vi "betav3 labview.vi"() -> ()   [LabVIEW 2016]
uses:
  <vilib>/Instr/_visa.llb/VISA Configure Serial Port (Instr).vi
panel:
  in  "Stop":bool
  out "Arduino connecté ?":bool
  in  "Port de communication":refnum<visa-resource-name>="COM4"
  in  "?":T1(tab)
  in  "Emplacement mémoire":string(combo)
  out "Données lue":string
  in  "Adresse de fin+1":string
  in  "Adresse de début":string
  in  "Données à écrire":string
  in  "Lecture":bool
  in  "Ecriture":bool
  in  "Lecture totale de l'EEPROM":bool
  out "Commentaire 2":string
  out "Board serial number":string
  out "Code article":string
  out "Test sonde mobile":string
  out "Test synor":string
  out "Test ICT":string
  out "Test FCT1":string
  out "Test ESS":string
  out "Test FCT2":string
  out "Version soft 1":string
  out "Version soft 2":string
  out "Commentaires 1":string
  out "Version soft 3":string
  out "Mapping":string
  # "Programmateur EEPROM beta v2"
  # "Programmateur EEPROM"
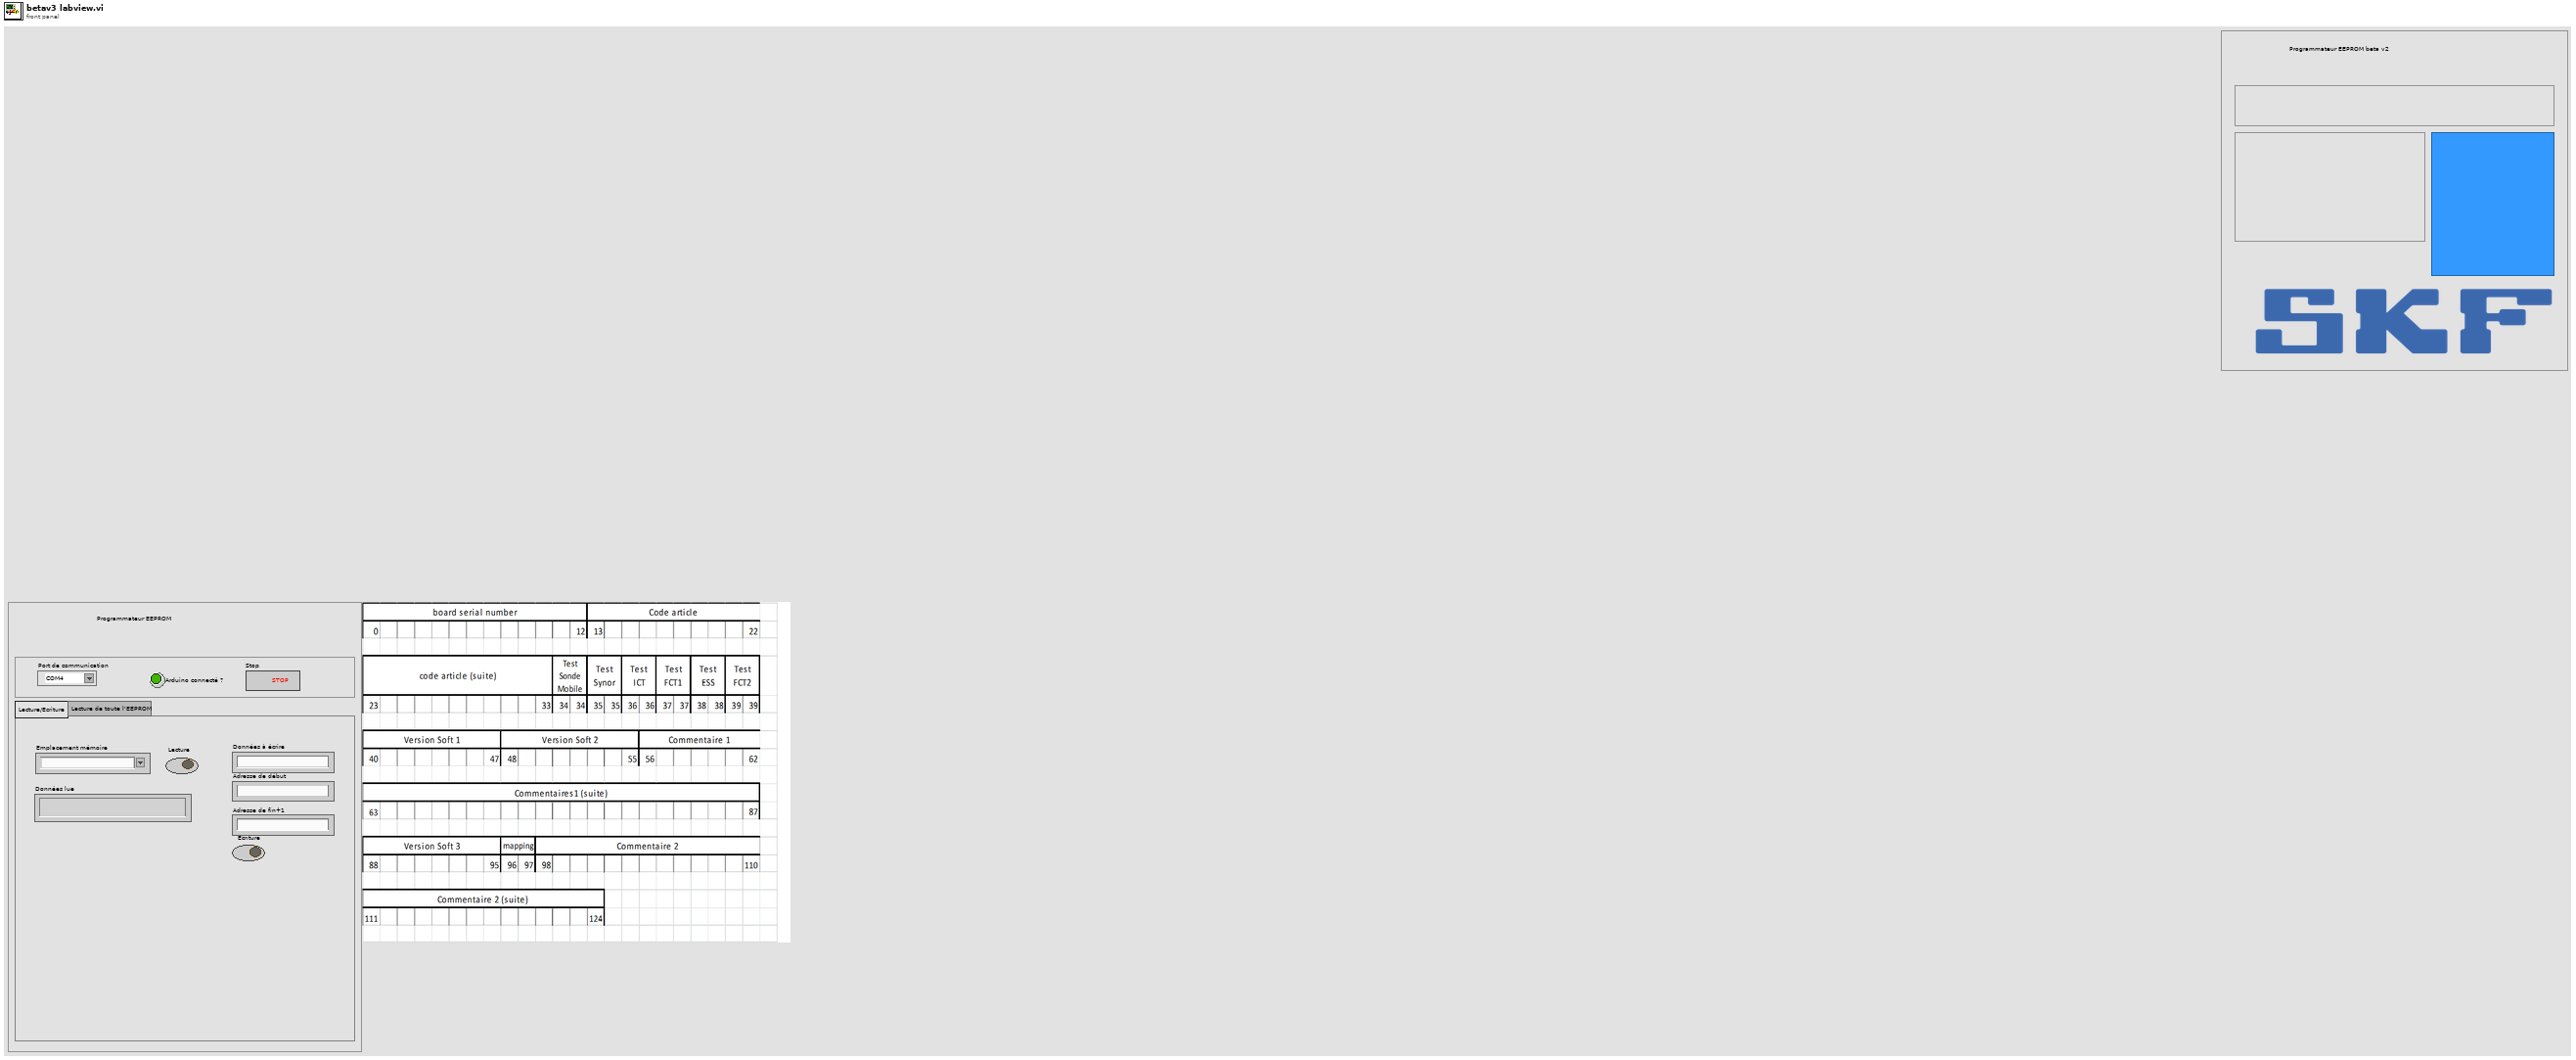
[diagram p1: front panel]
types:
  T1 = enum32{"Lecture/Ecriture", "Lecture de toute l'EEPROM"}
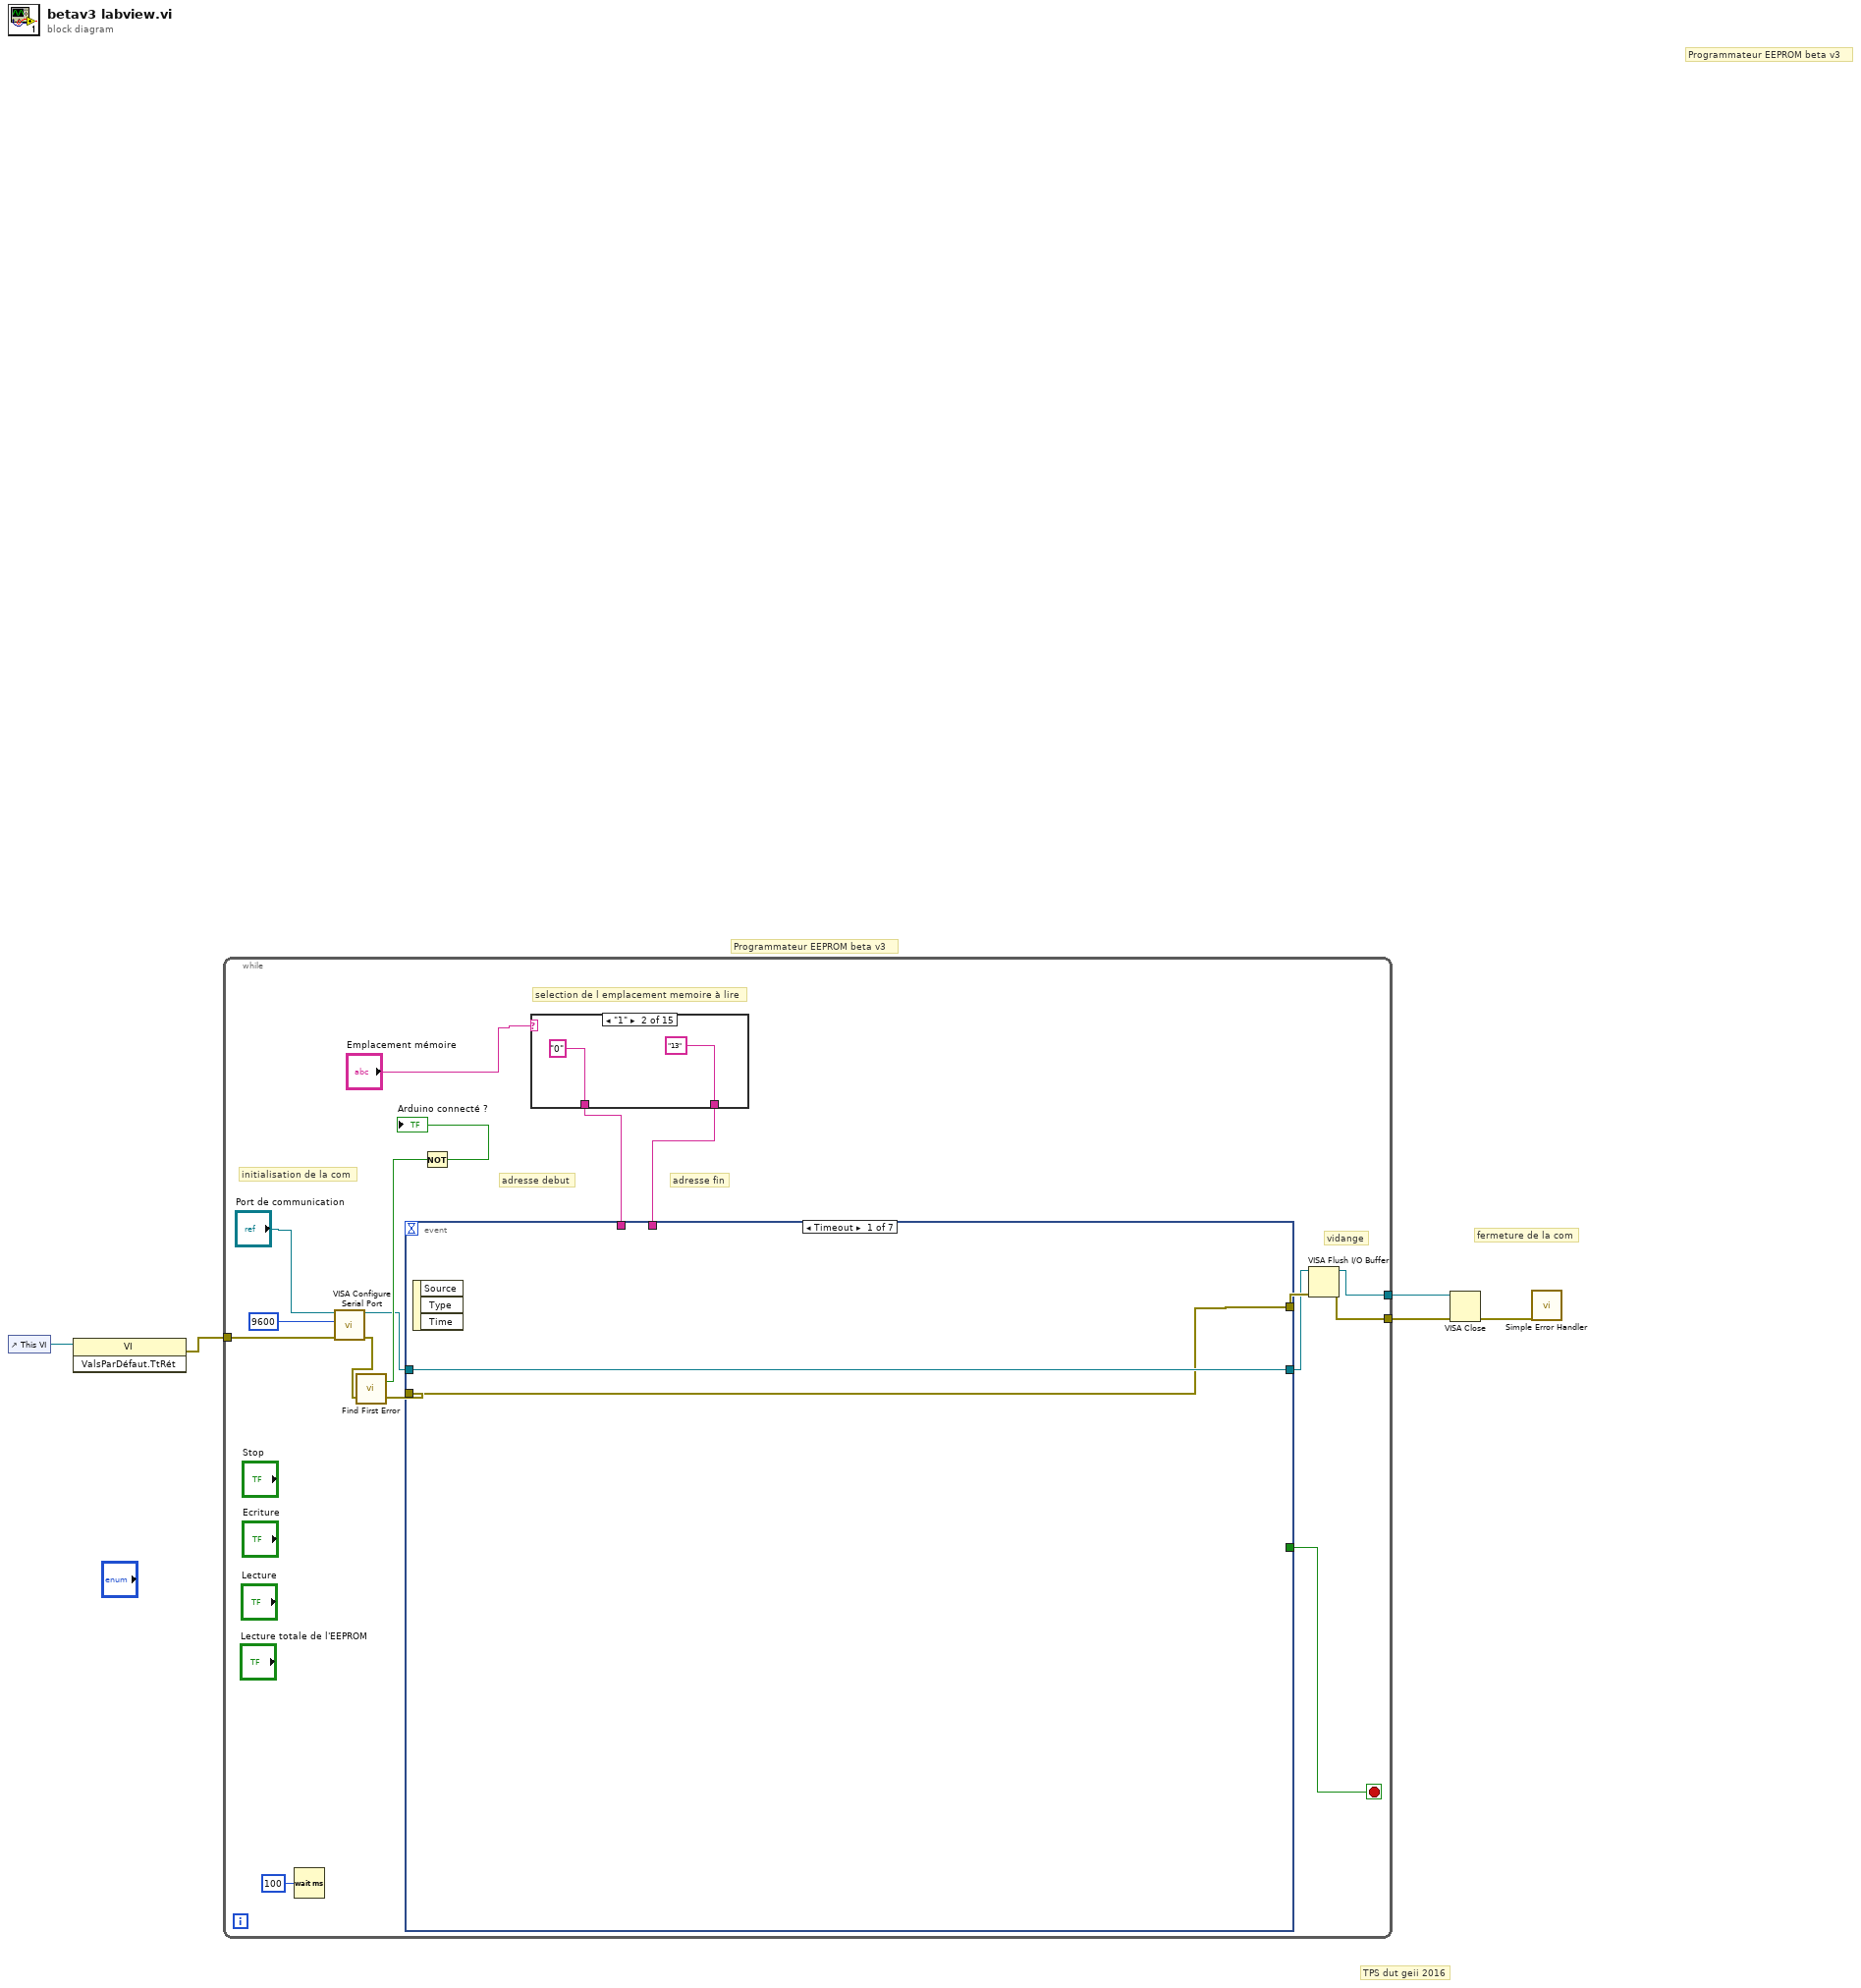
[diagram p0: block diagram]
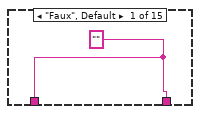
[diagram p2: hidden frame]
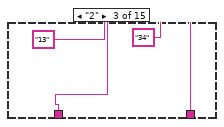
[diagram p3: hidden frame]
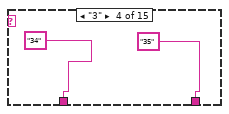
[diagram p4: hidden frame]
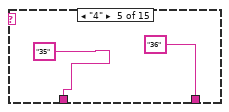
[diagram p5: hidden frame]
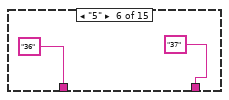
[diagram p6: hidden frame]
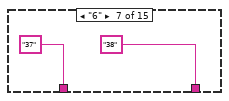
[diagram p7: hidden frame]
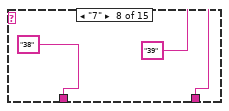
[diagram p8: hidden frame]
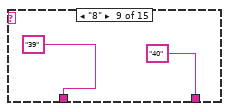
[diagram p9: hidden frame]
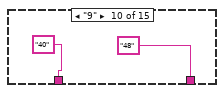
[diagram p10: hidden frame]
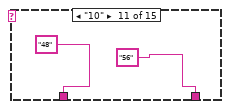
[diagram p11: hidden frame]
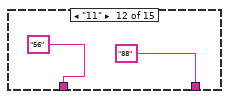
[diagram p12: hidden frame]
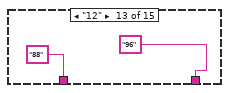
[diagram p13: hidden frame]
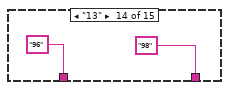
[diagram p14: hidden frame]
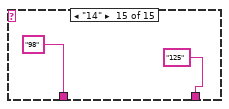
[diagram p15: hidden frame]
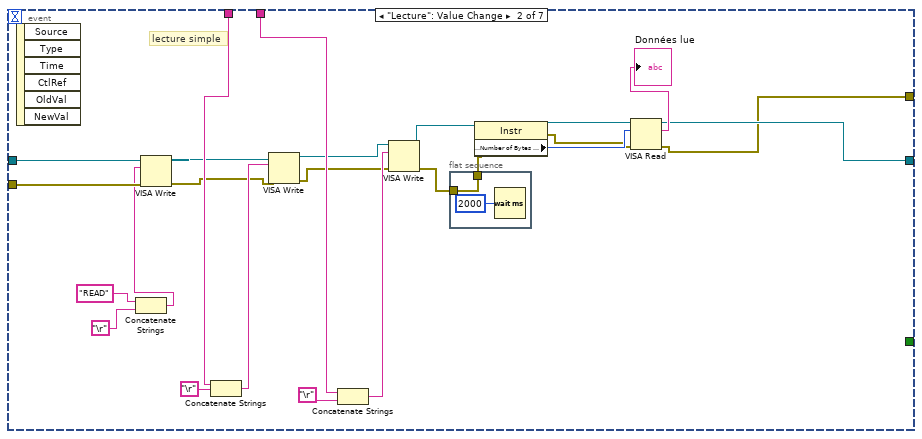
[diagram p16: hidden frame]
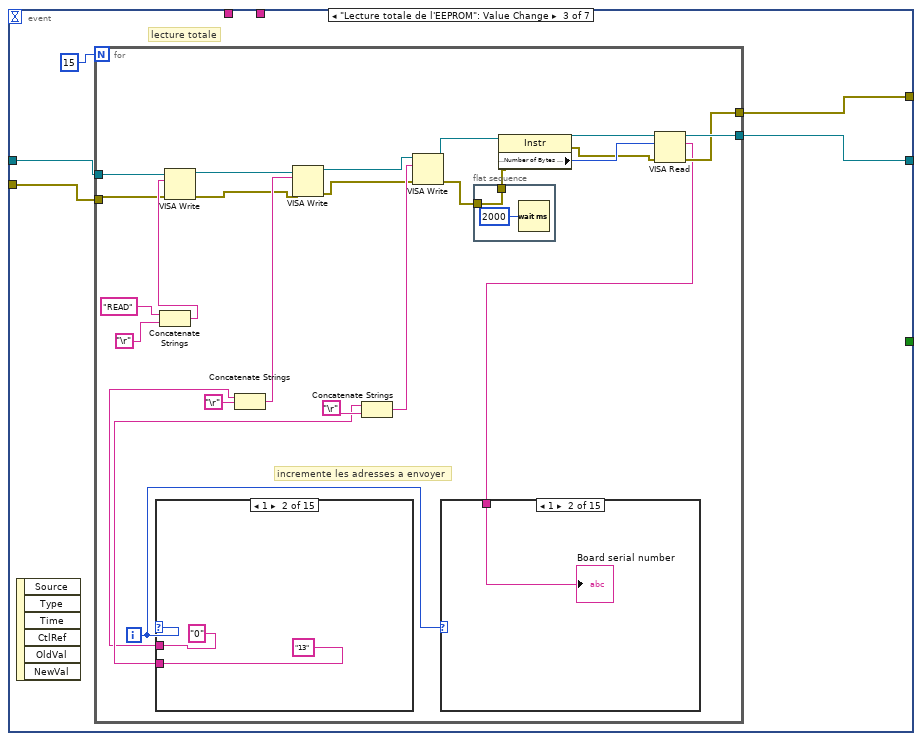
[diagram p17: hidden frame]
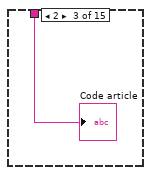
[diagram p19: hidden frame]
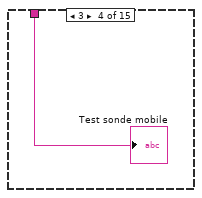
[diagram p20: hidden frame]
diagram:
  # "fermeture de la com"
  # "TPS dut geii 2016"
  # "Programmateur EEPROM beta v3"
  # "Programmateur EEPROM beta v3"
  n1 = control-ref of="This VI"() -> (w4:refnum<vi>)
  n2 = invoke class="VI" method="ValsParDéfaut.TtRét"(reference=w4) -> (error out=w1:errorcluster)  [unwired: 2 in, 2 out]
  n3 = while {
    tunnel: [w17] -> w5
    tunnel: [w16] -> w3
    tunnel: w1 -> [w15]
    stop <- w8 stop-if-true
    # "vidange"
    # "selection de l emplacement memoire à lire"
    # "initialisation de la com"
    # "adresse fin"
    # "adresse debut"
    n4 = Wait (ms)(milliseconds to wait=u32 100 ("attente (ms)")) -> ()  [unwired: 1 out]
    n5 = call-poly "VISA Configure Serial Port"("VISA resource name"="Port de communication", "baud rate (9600)"=u32 9600, "error in (no error)"=w15) -> ("VISA resource name out"=w13:refnum<visa-resource-name>, "error out"=w14:errorcluster)  [unwired: 11 in]
    n6 = call <vilib>:"Find First Error.vi"("error in (no error)"=w14) -> ("error out"=w18:errorcluster, "error?"=w19:bool)  [unwired: 3 in]
    n7 = Not(x=w19) -> (.not. x?=→"Arduino connecté ?":bool)
    n8 = case shown="\"1\"" "Emplacement mémoire" {
      tunnel: [w23 "0" "13" "34" "35" "36" "37" "38" "39" "40" "48" "56" "88" "96" "98"] -> w10
      tunnel: [w23 "13" "34" "35" "36" "37" "38" "39" "40" "48" "56" "88" "96" "98" "125"] -> w9
      frame "Faux", Default {
        w23 = ""
      }
      frame "1" {
      }
      frame "2" {
      }
      frame "3" {
      }
      frame "4" {
      }
      frame "5" {
      }
      frame "6" {
      }
      frame "7" {
      }
      frame "8" {
      }
      frame "9" {
      }
      frame "10" {
      }
      frame "11" {
      }
      frame "12" {
      }
      frame "13" {
      }
      frame "14" {
      }
    }
    n9 = event shown="[0] Timeout" {
      selector: _ -> [_ _ _ _ _ _ _]
      dyn-events: _ -> [_ _ _ _ _ _ _]
      timeout: _ -> [_ _ _ _ _ _ _]
      tunnel: w13 -> [w53 w77 w84 w155 w157 w159 w170]
      tunnel: w10 -> [_ w76 _ _ _ _ _]
      tunnel: w9 -> [_ w75 _ _ _ _ _]
      tunnel: w18 -> [w52 w74 w83 w156 w158 w160 w169]
      tunnel: [_ _ _ _ _ TRUE _] -> w8
      tunnel: [w53 w55 w82 w155 w157 w159 w164] -> w6
      tunnel: [w52 w54 w81 w156 w158 w160 w162] -> w7
      event Timeout {
        n10 = event-data() -> ()  [unwired: 1 in, 3 out]
      }
      event "Lecture": Value Change {
        # "lecture simple"
        n11 = event-data() -> ()  [unwired: 1 in, 6 out]
        n12 = Concatenate Strings("READ", "\r") -> (w70:string)
        n13 = VISA Write(VISA resource name=w77, write buffer=w70, error in (no error)=w74) -> (VISA resource name out=w69:refnum<visa-resource-name>, error out=w60:errorcluster)  [unwired: 1 out]
        n14 = Concatenate Strings(w76, "\r") -> (w67:string)
        n15 = VISA Write(VISA resource name=w69, write buffer=w67, error in (no error)=w60) -> (VISA resource name out=w66:refnum<visa-resource-name>, error out=w59:errorcluster)  [unwired: 1 out]
        n16 = Concatenate Strings(w75, "\r") -> (w64:string)
        n17 = VISA Write(VISA resource name=w66, write buffer=w64, error in (no error)=w59) -> (VISA resource name out=w61:refnum<visa-resource-name>, error out=w56:errorcluster)  [unwired: 1 out]
        n18 = flat-sequence {
          tunnel: [w78] -> w57
          tunnel: w56 -> [w78]
          frame #0 {
            n19 = Wait (ms)(milliseconds to wait=u32 2000 ("attente (ms)")) -> ()  [unwired: 1 out]
          }
        }
        n20 = property class="Instr"(reference=w61, error in=w57) -> (reference out=w62:refnum<visa-resource-name>, error out=w58:errorcluster, "Serial Settings:Number of Bytes at Serial Port"=w63:u32)
        n21 = VISA Read(VISA resource name=w62, byte count=w63, error in (no error)=w58) -> (VISA resource name out=w55:refnum<visa-resource-name>, read buffer=→"Données lue":string, error out=w54:errorcluster)  [unwired: 1 out]
      }
      event "Lecture totale de l'EEPROM": Value Change {
        # "lecture totale"
        n22 = event-data() -> ()  [unwired: 1 in, 6 out]
        n23 = for {
          N: 15 ("x") -> [_]
          tunnel: w84 -> [w91]
          tunnel: w83 -> [w92]
          tunnel: [w90] -> w82
          tunnel: [w89] -> w81
          i -> [w86]
          # "incremente les adresses a envoyer"
          n24 = case shown="1" w86 {
            tunnel: [w126 "13" "34" "35" "36" "37" "38" "39" "40" "48" "56" "88" "96" "98" "125"] -> w88
            tunnel: [w126 "0" "13" "34" "35" "36" "37" "38" "39" "40" "48" "56" "88" "96" "98"] -> w87
            frame 0, Default {
              w126 = ""
            }
            frame 1 {
            }
            frame 2 {
            }
            frame 3 {
            }
            frame 4 {
            }
            frame 5 {
            }
            frame 6 {
            }
            frame 7 {
            }
            frame 8 {
            }
            frame 9 {
            }
            frame 10 {
            }
            frame 11 {
            }
            frame 12 {
            }
            frame 13 {
            }
            frame 14 {
            }
          }
          n25 = Concatenate Strings("READ", "\r") -> (w107:string)
          n26 = VISA Write(VISA resource name=w91, write buffer=w107, error in (no error)=w92) -> (VISA resource name out=w106:refnum<visa-resource-name>, error out=w97:errorcluster)  [unwired: 1 out]
          n27 = Concatenate Strings(w87, "\r") -> (w104:string)
          n28 = VISA Write(VISA resource name=w106, write buffer=w104, error in (no error)=w97) -> (VISA resource name out=w103:refnum<visa-resource-name>, error out=w96:errorcluster)  [unwired: 1 out]
          n29 = Concatenate Strings(w88, "\r") -> (w101:string)
          n30 = VISA Write(VISA resource name=w103, write buffer=w101, error in (no error)=w96) -> (VISA resource name out=w98:refnum<visa-resource-name>, error out=w93:errorcluster)  [unwired: 1 out]
          n31 = flat-sequence {
            tunnel: [w124] -> w94
            tunnel: w93 -> [w124]
            frame #0 {
              n32 = Wait (ms)(milliseconds to wait=u32 2000 ("attente (ms)")) -> ()  [unwired: 1 out]
            }
          }
          n33 = property class="Instr"(reference=w98, error in=w94) -> (reference out=w99:refnum<visa-resource-name>, error out=w95:errorcluster, "Serial Settings:Number of Bytes at Serial Port"=w100:u32)
          n34 = VISA Read(VISA resource name=w99, byte count=w100, error in (no error)=w95) -> (VISA resource name out=w90:refnum<visa-resource-name>, read buffer=w85:string, error out=w89:errorcluster)  [unwired: 1 out]
          n35 = case shown="1" w86 {
            tunnel: w85 -> [_ w110 w111 w112 w113 w114 w115 w116 w117 w118 w119 w120 w121 w122 w123]
            frame 0, Default {
            }
            frame 1 {
              "Board serial number" <- w110
            }
            frame 2 {
              "Code article" <- w111
            }
            frame 3 {
              "Test sonde mobile" <- w112
            }
            frame 4 {
              "Test synor" <- w113
            }
            frame 5 {
              "Test ICT" <- w114
            }
            frame 6 {
              "Test FCT1" <- w115
            }
            frame 7 {
              "Test ESS" <- w116
            }
            frame 8 {
              "Test FCT2" <- w117
            }
            frame 9 {
              "Version soft 1" <- w118
            }
            frame 10 {
              "Version soft 2" <- w119
            }
            frame 11 {
              "Commentaires 1" <- w120
            }
            frame 12 {
              "Version soft 3" <- w121
            }
            frame 13 {
              "Mapping" <- w122
            }
            frame 14 {
              "Commentaire 2" <- w123
            }
          }
        }
      }
      event "Port de communication": Value Change {
        n36 = event-data() -> ()  [unwired: 1 in, 6 out]
      }
      event "Emplacement mémoire": Value Change {
        n37 = event-data() -> ()  [unwired: 1 in, 6 out]
      }
      event "Stop": Value Change {
        n38 = event-data() -> ()  [unwired: 1 in, 6 out]
      }
      event "Ecriture": Value Change {
        # "test"
        n39 = event-data() -> ()  [unwired: 1 in, 6 out]
        n40 = Concatenate Strings("WRITE", "\r") -> (w174:string)
        n41 = VISA Write(VISA resource name=w170, write buffer=w174, error in (no error)=w169) -> (VISA resource name out=w178:refnum<visa-resource-name>, error out=w168:errorcluster)  [unwired: 1 out]
        n42 = Wait (ms)(milliseconds to wait=u32 100 ("attente (ms)")) -> ()  [unwired: 1 out]
        n43 = Concatenate Strings("Données à écrire", "\r") -> (w175:string)
        n44 = VISA Write(VISA resource name=w178, write buffer=w175, error in (no error)=w168) -> (VISA resource name out=w179:refnum<visa-resource-name>, error out=w167:errorcluster)  [unwired: 1 out]
        n45 = Concatenate Strings("Adresse de début", "\r") -> (w181:string)
        n46 = VISA Write(VISA resource name=w179, write buffer=w181, error in (no error)=w167) -> (VISA resource name out=w185:refnum<visa-resource-name>, error out=w166:errorcluster)  [unwired: 1 out]
        n47 = Concatenate Strings("Adresse de fin+1", "\r") -> (w171:string)
        n48 = VISA Write(VISA resource name=w185, write buffer=w171, error in (no error)=w166) -> (VISA resource name out=w164:refnum<visa-resource-name>, error out=w163:errorcluster)  [unwired: 1 out]
        n49 = flat-sequence {
          tunnel: [w186] -> w162
          tunnel: w163 -> [w186]
          frame #0 {
            n50 = Wait (ms)(milliseconds to wait=u32 1000 ("attente (ms)")) -> ()  [unwired: 1 out]
          }
        }
      }
    }
    n51 = VISA Flush I/O Buffer(VISA resource name=w6, error in (no error)=w7) -> (VISA resource name out=w17:refnum<visa-resource-name>, error out=w16:errorcluster)  [unwired: 1 in]
  }
  n52 = VISA Close(VISA resource name=w5, error in (no error)=w3) -> (error out=w2:errorcluster)
  n53 = call <vilib>:"Simple Error Handler.vi"("error in (no error)"=w2) -> ()  [unwired: 4 in, 5 out]
